vi "Configure List Steps.vi"(0 "VISA resource name":refnum<visa-resource-name>, 1 "List Step Voltage":T1 {"End DC Voltage (0 V)" format="%.3g"; "End AC Voltage (0 V)" format="%.3g"; "Start DC Voltage (0 V)" format="%.3g"; "Start AC Voltage (0 V)" format="%.3g"}, 2 "Step Number (0)":u32 max=99 step=1, 5 "Start Frequency (50 Hz)":dbl=50.0 min=43.0 max=1200.0 format="%.3g", 7 "End Frequency (50 Hz)":dbl=50.0 min=43.0 max=1200.0 format="%.3g", 9 "List Step Time Cycle (1 ms/cycles)":u32=1 min=1 max=100000, 11 "error in (no error)":errorcluster, 12 "List Step Count (0)":u32 max=200 step=1) -> (4 "VISA resource name out":refnum<visa-resource-name>, 15 "error out":errorcluster)   [LabVIEW 2018, in "BK Precision 983X Series.lvlib"]
doc: "Configures the list step parameters: Start and end AC and DC voltage, start and end frequency, time/cycle, step count.\n\nNote: Recall a list first using <b>Save Recall List Program.vi</b> before running this vi. Otherwise, steps will not be saved."
uses:
  <instrlib>/BK Precision 983X Series/BK Precision 983X Series.lvlib
panel:
  # "V"
  # "V"
  # "V"
  # "V"
  # "Hz"
  # "Hz"
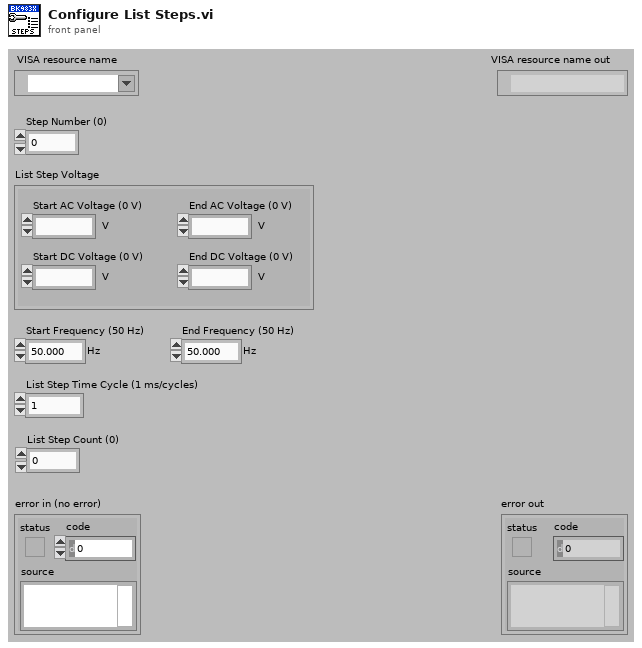
[diagram p1: front panel]
types:
  T1 = cluster{"Start AC Voltage (0 V)":dbl, "Start DC Voltage (0 V)":dbl, "End AC Voltage (0 V)":dbl, "End DC Voltage (0 V)":dbl}
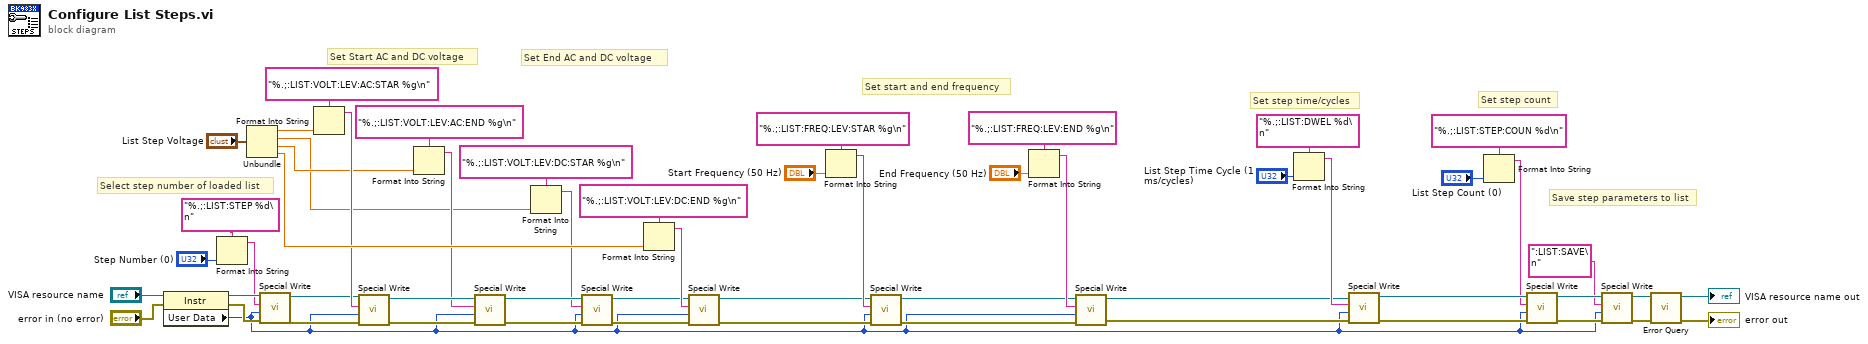
[diagram p0: block diagram]
diagram:
  # "Set step count"
  # "Set step time/cycles"
  # "Set start and end frequency"
  # "Set End AC and DC voltage"
  # "Set Start AC and DC voltage"
  # "Select step number of loaded list"
  # "Save step parameters to list"
  n1 = property class="Instr"(reference="VISA resource name", error in="error in (no error)") -> (reference out=w35:refnum<visa-resource-name>, error out=w34:errorcluster, "User Data"=w2:u32)
  n2 = Format Into String(format string="%.;:LIST:STEP %d\n", "Step Number (0)") -> (resulting string=w33:string)  [unwired: 2 in, 1 out]
  n3 = Unbundle("List Step Voltage") -> ("Start AC Voltage (0 V)"=w48:dbl, "Start DC Voltage (0 V)"=w8:dbl, "End AC Voltage (0 V)"=w9:dbl, "End DC Voltage (0 V)"=w44:dbl)
  n4 = call <instrlib>:"Special Write.vi"("error in (no error)"=w34, "Delay (0 ms)"=w2, "Input String"=w33, "VISA resource name"=w35) -> ("error out"=w30:errorcluster, "VISA resource name out"=w31:refnum<visa-resource-name>)  [unwired: 6 in]
  n5 = Format Into String(format string="%.;:LIST:VOLT:LEV:AC:STAR %g\n", w48) -> (resulting string=w32:string)  [unwired: 2 in, 1 out]
  n6 = call <instrlib>:"Special Write.vi"("error in (no error)"=w30, "Delay (0 ms)"=w2, "Input String"=w32, "VISA resource name"=w31) -> ("error out"=w28:errorcluster, "VISA resource name out"=w29:refnum<visa-resource-name>)  [unwired: 6 in]
  n7 = Format Into String(format string="%.;:LIST:VOLT:LEV:AC:END %g\n", w9) -> (resulting string=w10:string)  [unwired: 2 in, 1 out]
  n8 = call <instrlib>:"Special Write.vi"("error in (no error)"=w28, "Delay (0 ms)"=w2, "Input String"=w10, "VISA resource name"=w29) -> ("error out"=w26:errorcluster, "VISA resource name out"=w27:refnum<visa-resource-name>)  [unwired: 6 in]
  n9 = Format Into String(format string="%.;:LIST:VOLT:LEV:DC:STAR %g\n", w8) -> (resulting string=w7:string)  [unwired: 2 in, 1 out]
  n10 = call <instrlib>:"Special Write.vi"("error in (no error)"=w26, "Delay (0 ms)"=w2, "Input String"=w7, "VISA resource name"=w27) -> ("error out"=w23:errorcluster, "VISA resource name out"=w24:refnum<visa-resource-name>)  [unwired: 6 in]
  n11 = Format Into String(format string="%.;:LIST:VOLT:LEV:DC:END %g\n", w44) -> (resulting string=w25:string)  [unwired: 2 in, 1 out]
  n12 = call <instrlib>:"Special Write.vi"("error in (no error)"=w23, "Delay (0 ms)"=w2, "Input String"=w25, "VISA resource name"=w24) -> ("error out"=w20:errorcluster, "VISA resource name out"=w21:refnum<visa-resource-name>)  [unwired: 6 in]
  n13 = Format Into String(format string="%.;:LIST:FREQ:LEV:STAR %g\n", "Start Frequency (50 Hz)") -> (resulting string=w22:string)  [unwired: 2 in, 1 out]
  n14 = call <instrlib>:"Special Write.vi"("error in (no error)"=w20, "Delay (0 ms)"=w2, "Input String"=w22, "VISA resource name"=w21) -> ("error out"=w17:errorcluster, "VISA resource name out"=w18:refnum<visa-resource-name>)  [unwired: 6 in]
  n15 = Format Into String(format string="%.;:LIST:FREQ:LEV:END %g\n", "End Frequency (50 Hz)") -> (resulting string=w19:string)  [unwired: 2 in, 1 out]
  n16 = call <instrlib>:"Special Write.vi"("error in (no error)"=w17, "Delay (0 ms)"=w2, "Input String"=w19, "VISA resource name"=w18) -> ("error out"=w14:errorcluster, "VISA resource name out"=w15:refnum<visa-resource-name>)  [unwired: 6 in]
  n17 = Format Into String(format string="%.;:LIST:DWEL %d\n", "List Step Time Cycle (1 ms/cycles)") -> (resulting string=w16:string)  [unwired: 2 in, 1 out]
  n18 = call <instrlib>:"Special Write.vi"("error in (no error)"=w14, "Delay (0 ms)"=w2, "Input String"=w16, "VISA resource name"=w15) -> ("error out"=w12:errorcluster, "VISA resource name out"=w13:refnum<visa-resource-name>)  [unwired: 6 in]
  n19 = Format Into String(format string="%.;:LIST:STEP:COUN %d\n", "List Step Count (0)") -> (resulting string=w11:string)  [unwired: 2 in, 1 out]
  n20 = call <instrlib>:"Special Write.vi"("error in (no error)"=w12, "Delay (0 ms)"=w2, "Input String"=w11, "VISA resource name"=w13) -> ("error out"=w4:errorcluster, "VISA resource name out"=w3:refnum<visa-resource-name>)  [unwired: 6 in]
  n21 = call <instrlib>:"Special Write.vi"("error in (no error)"=w4, "Delay (0 ms)"=w2, "Input String"=":LIST:SAVE\n", "VISA resource name"=w3) -> ("error out"=w5:errorcluster, "VISA resource name out"=w6:refnum<visa-resource-name>)  [unwired: 6 in]
  n22 = call <instrlib>:"Error Query.vi"("error in (no error)"=w5, "VISA resource name"=w6) -> ("error out"=→"error out":errorcluster, "VISA resource name out"=→"VISA resource name out":refnum<visa-resource-name>)  [unwired: 6 in, 2 out]
